vi "nifxpmath_DiscreteDelay_ScriptedToCoerceScalar.vi"() -> (3 "numeric":fxp<+/-,16,8> format="%.6f")   [LabVIEW 2017]
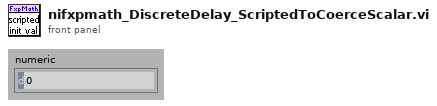
[diagram p1: front panel]
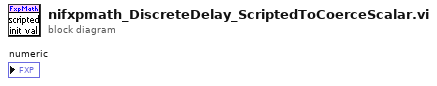
[diagram p0: block diagram]
diagram:
